vi "Create DC Power Session.vi"(8 "error in (no error)":errorcluster, 10 "gRPC device server location":T1, 11 "session information":T2) -> (0 "error out":errorcluster, 3 "instrument handle":refnum<k15>)   [LabVIEW 2020, in "NIDCPowerSourceDCVoltage.lvlib"]
doc: "Creates and returns an gRPC based NI DC power instrument handle."
uses:
  NIDCPowerSourceDCVoltage.lvlib
  <vilib>/MeasurementLink/MeasurementLink Session Management Client/RPC Messages/ni_measurementlink_sessionmanagement_v1_SessionInformation.ctl
  <vilib>/MeasurementLink/MeasurementLink Session Management Client/RPC Messages/nidevice_grpc_Session.ctl
  <vilib>/MeasurementLink/MeasurementLink Session Management Client/RPC Messages/ni_measurementlink_sessionmanagement_v1_ChannelMapping.ctl
  <vilib>/MeasurementLink/MeasurementLink Discovery Client/RPC Messages/ni_measurementlink_discovery_v1_ServiceLocation.ctl
  <vilib>/MeasurementLink/MeasurementLink Session Management Client/MeasurementLink Session Management Client.lvlib
  <vilib>/MeasurementLink/MeasurementLink Discovery Client/MeasurementLink Discovery Client.lvlib
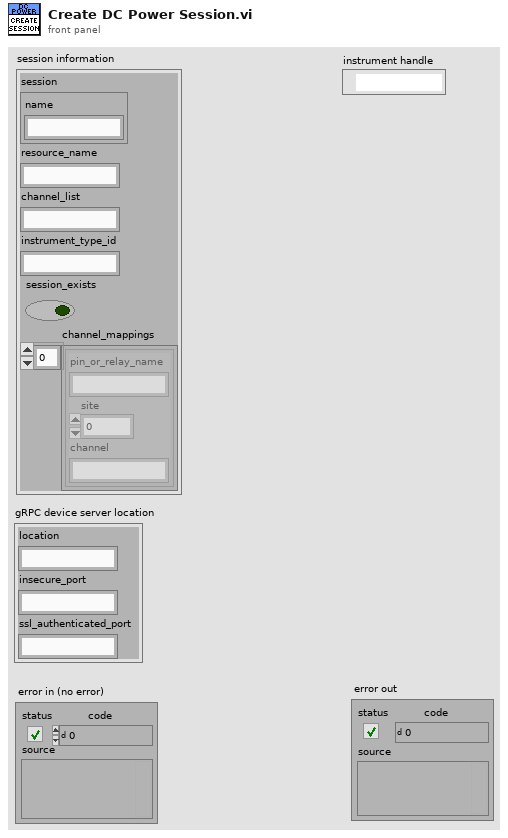
[diagram p1: front panel]
types:
  T1 = typedef "MeasurementLink Discovery Client.lvlib/ni_measurementlink_discovery_v1_ServiceLocation.ctl" = cluster{"location":string, "insecure_port":string, "ssl_authenticated_port":string}
  T2 = typedef "MeasurementLink Session Management Client.lvlib/ni_measurementlink_sessionmanagement_v1_SessionInformation.ctl" = cluster{"session":T3, "resource_name":string, "channel_list":string, "instrument_type_id":string, "session_exists":bool, "channel_mappings":T4[]}
  T3 = typedef "MeasurementLink Session Management Client.lvlib/nidevice_grpc_Session.ctl" = cluster{"name":string}
  T4 = typedef "MeasurementLink Session Management Client.lvlib/ni_measurementlink_sessionmanagement_v1_ChannelMapping.ctl" = cluster{"pin_or_relay_name":string, "site":i32, "channel":string}
  T5 = typedef "niDCPower gRPC Device Server.ctl" = cluster{"session name":string, "address (localhost)":string, "port (31763)":u32}
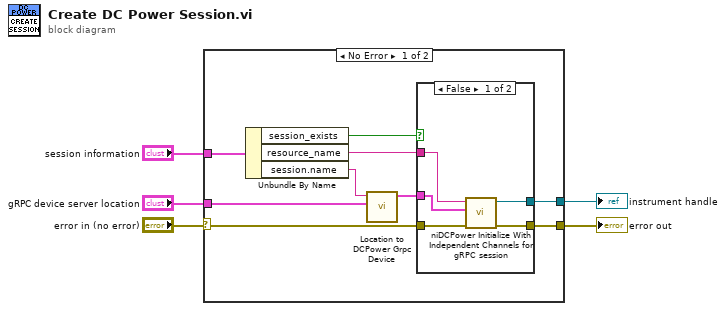
[diagram p0: block diagram]
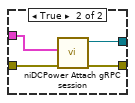
[diagram p2: hidden frame]
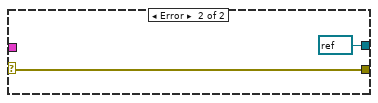
[diagram p3: hidden frame]
diagram:
  n1 = case shown="No Error" "error in (no error)" {
    selector: "error in (no error)" -> [w6 w25]
    tunnel: "session information" -> [w14 _]
    tunnel: "gRPC device server location" -> [w11 _]
    tunnel: [w8 w25] -> w3
    tunnel: [w7 refnum<k15> refnum ("instrument handle out")] -> w2
    frame No Error {
      n2 = Unbundle By Name(w14) -> ("session_exists"=w13:bool, "resource_name"=w9:string, "session.name"=w12:string)
      n3 = call "Location to DCPower Grpc Device.vi"("Grpc Device Location"=w11, "Session Name"=w12) -> ("NI gRPC Device Server Out"=w10:T5)  [unwired: 9 in]
      n4 = case shown="False" w13 {
        tunnel: w10 -> [w17 w21]
        tunnel: w9 -> [w16 _]
        tunnel: w6 -> [w19 w23]
        tunnel: [w18 w22] -> w8
        tunnel: [w15 w20] -> w7
        frame False {
          n5 = call <instrlib>:"niDCPower Initialize With Independent Channels for gRPC session.vi"("error in (no error)"=w19, "gRPC options"=w17, "resource name"=w16) -> ("error out"=w18:errorcluster, "instrument handle out"=w15:refnum<k15>)  [unwired: 7 in]
        }
        frame True {
          n6 = call <instrlib>:"niDCPower Attach gRPC session.vi"("error in (no error)"=w23, "gRPC options"=w21) -> ("error out"=w22:errorcluster, "instrument handle out"=w20:refnum<k15>)  [unwired: 8 in]
        }
      }
    }
    frame Error {
    }
  }
  "instrument handle" <- w2
  "error out" <- w3
